vi "Build Attr ID.vi"(10 "Attr Name":string, 11 "Unique ID":string) -> (3 "Attr ID Out":string)   [LabVIEW 2017, in "Tree API.lvlib" / "Tree.lvclass"]
uses:
  Tree.lvclass
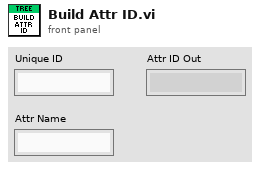
[diagram p1: front panel]
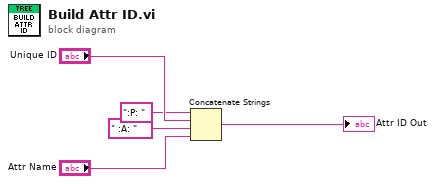
[diagram p0: block diagram]
diagram:
  n1 = Concatenate Strings(":P: " ("string"), "Unique ID", " :A: " ("string"), "Attr Name") -> (→"Attr ID Out":string)
